vi "Timing.Iteration.Increment.vi"(11 "Timing in":refnum<class "Timing.lvclass">) -> (3 "Timing out":refnum<class "Timing.lvclass">)   [LabVIEW 2017, in "DSF Core.lvlib" / "Timing.lvclass"]
uses:
  Timing.lvclass
  Timing.lvclass/Timing.ctl
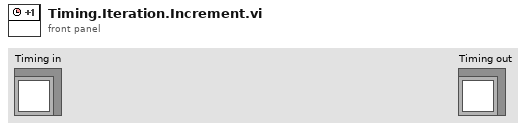
[diagram p1: front panel]
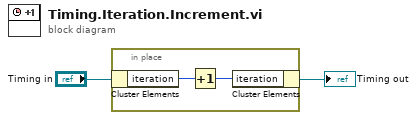
[diagram p0: block diagram]
diagram:
  n1 = in-place {
    n2 = in-place-cluster #1("Timing in") -> ("iteration"=w4:u64)
    n3 = Increment(x=w4) -> (x+1=w3:u64)
    n4 = in-place-cluster #1("iteration"=w3) -> (→"Timing out":refnum<class "Timing.lvclass">)
  }
